vi "configRead.vi"(10 "Self":T1={"refDes"="ERR000", "IP"="localhost", "DI"=0, "DO"=0, "AI"=0, "AO"=0, "Description"="ERR", "TC"=0, "channelDefinitions"=[]}, 11 "configPath":path=path "C:/Users/miles/OneDrive - Embry-Riddle Aeronautical University/Admin/Facilities/TC3/TC3 DAC/Code/Sandbox/Node based/controlNode/Configuration/nodeConfig_0.xlsx") -> (2 "Self":T1={"refDes"="ERR000", "IP"="localhost", "DI"=0, "DO"=0, "AI"=0, "AO"=0, "Description"="ERR", "TC"=0, "channelDefinitions"=[]}, 3 "Cancel/Err":bool)   [LabVIEW 2024]
uses:
  controls/self.ctl
  controls/channelDefinition.ctl
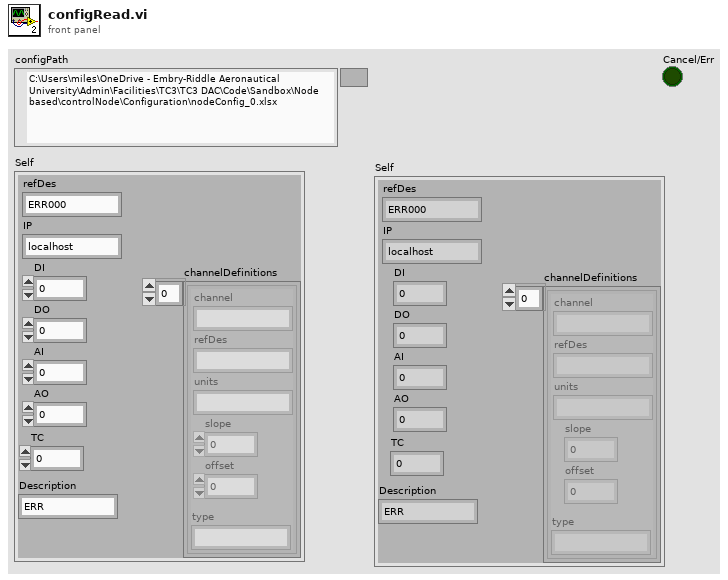
[diagram p1: front panel]
types:
  T1 = typedef "self.ctl" = cluster{"refDes":string, "IP":string, "DI":i32, "DO":i32, "AI":i32, "AO":i32, "Description":string, "TC":i32, "channelDefinitions":T2[]}
  T2 = typedef "channelDefinition.ctl" = cluster{"channel":string, "refDes":string, "units":string, "slope":dbl, "offset":dbl, "type":string}
  T3 = cluster{"[0]":string, "[1]":string, "[2]":string, "[3]":string, "[4]":string, "[5]":string, "[6]":string, "[7]":string, "[8]":string}
  T4 = cluster{"[0]":i32, "[1]":i32, "[2]":i32, "[3]":i32, "[4]":i32, "[5]":i32, "[6]":i32, "[7]":i32, "[8]":i32}
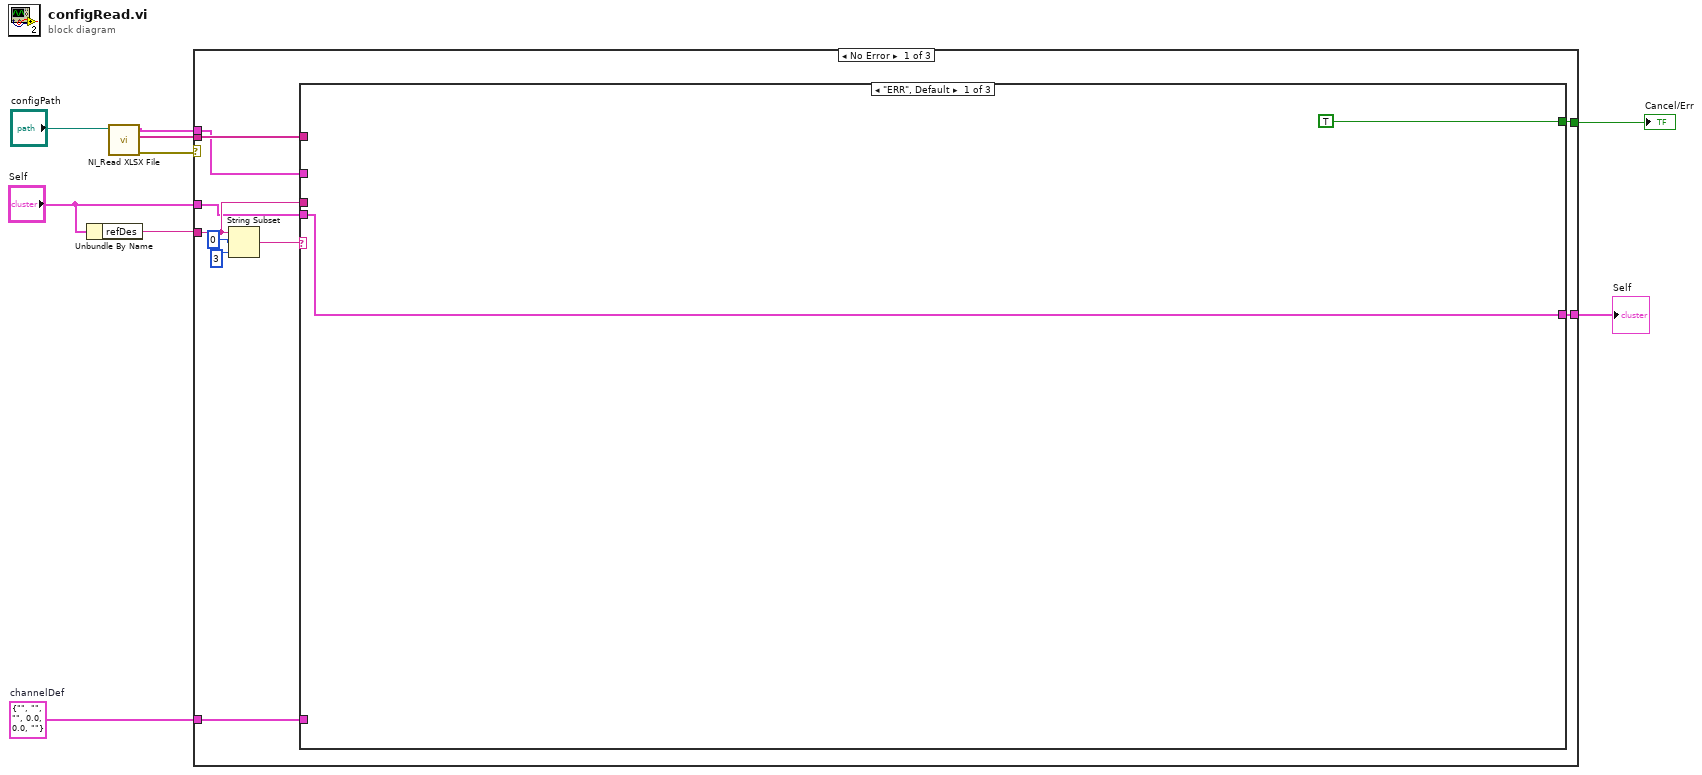
[diagram p0: block diagram]
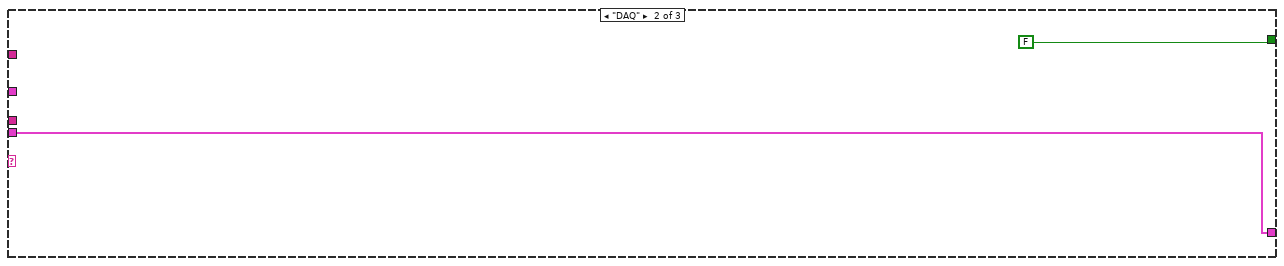
[diagram p2: hidden frame]
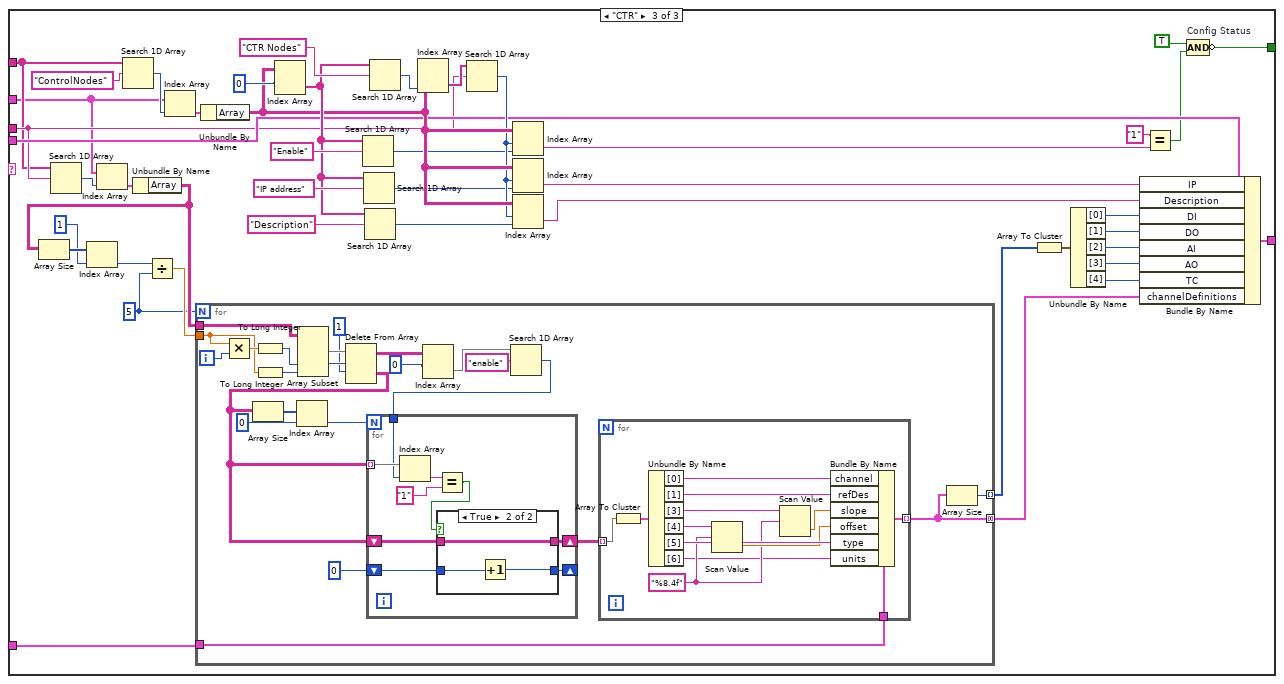
[diagram p3: hidden frame]
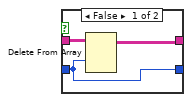
[diagram p4: hidden frame]
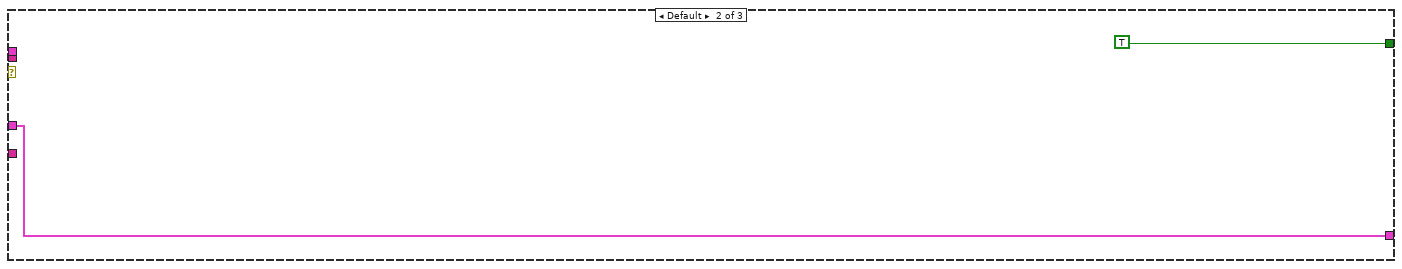
[diagram p5: hidden frame]
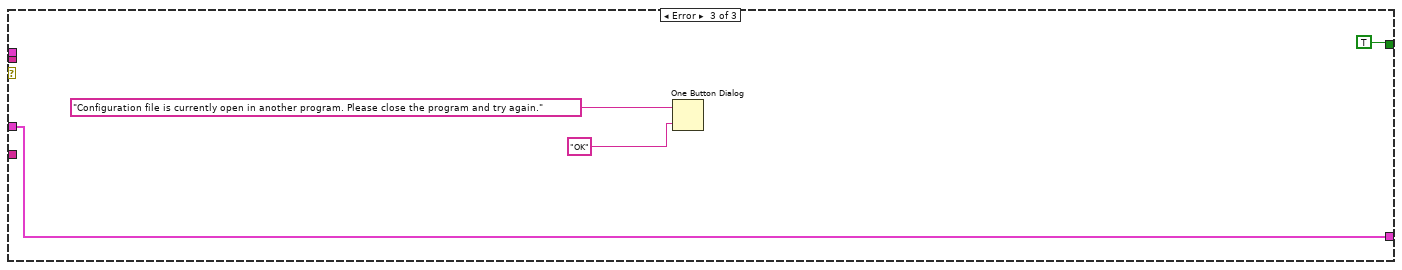
[diagram p6: hidden frame]
diagram:
  w1 = T2 {"channel"="", "refDes"="", "units"="", "slope"=0.0, "offset"=0.0, "type"=""}  # channelDef
  n1 = Unbundle By Name("Self") -> ("refDes"=w4:string)
  n2 = call "NI_Read XLSX File.vi"("XLSX File"="configPath") -> ("error out"=w8:errorcluster, "Sheet Names"=w7:string[], "Sheet Data"=w6:cluster{"Array":string[][]}[])  [unwired: 8 in]
  n3 = case shown="No Error" w8 {
    tunnel: [w13 TRUE TRUE] -> w9
    tunnel: w7 -> [w16 _ _]
    tunnel: w6 -> [w15 _ _]
    tunnel: w4 -> [w14 _ _]
    tunnel: "Self" -> [w12 w119 w123]
    tunnel: [w11 w119 w123] -> w2
    tunnel: w1 -> [w10 _ _]
    frame No Error {
      n4 = String Subset(string=w14, offset (0)=0, length (rest)=3 ("length (rest)")) -> (substring=w17:string)
      n5 = case shown="\"ERR\", Default" w17 {
        tunnel: w16 -> [_ _ w40]
        tunnel: w15 -> [_ _ w39]
        tunnel: w14 -> [_ _ w41]
        tunnel: [TRUE FALSE w60] -> w13
        tunnel: w12 -> [w20 w22 w50]
        tunnel: [w20 w22 w47] -> w11
        tunnel: w10 -> [_ _ w33]
        frame "ERR", Default {
        }
        frame "DAQ" {
        }
        frame "CTR" {
          w34 = 5 ("y")
          n6 = Search 1D Array(1D array=w40, element=w41) -> (index of element=w43:i32)  [unwired: 1 in]
          n7 = Index Array(array=w39, index=w43) -> (element=w42:cluster{"Array":string[][]})
          n8 = Search 1D Array(1D array=w40, element="ControlNodes") -> (index of element=w67:i32)  [unwired: 1 in]
          n9 = Unbundle By Name(w42) -> ("Array"=w38:string[][])
          n10 = Array Size(array=w38) -> (size(s)=w37:i32[])
          n11 = Index Array(array=w37, index=1) -> (element=w24:i32)
          n12 = Divide(x=w24, y=w34) -> (x/y=w35:dbl)
          n13 = Index Array(array=w39, index=w67) -> (element=w66:cluster{"Array":string[][]})
          n14 = for {
            N: w34 -> [_]
            tunnel: w38 -> [w90]
            tunnel: w35 -> [w88]
            tunnel: w33 -> [w78]
            tunnel: [w77] -> w25 mode=concatenating
            tunnel: [w76] -> w32 mode=indexing
            i -> [w75]
            n15 = Multiply(x=w88, y=w75) -> (x*y=w89:dbl)
            n16 = To Long Integer(number=w89) -> (32bit integer=w87:i32)
            n17 = To Long Integer(number=w88) -> (32bit integer=w85:i32)
            n18 = Array Subset(array=w90, index (col)=w87, length (col)=w85) -> (w86:string[][])  [unwired: 2 in]
            n19 = Delete From Array(array=w86, length=w85, index (row)=1) -> (deleted portion=w80:string[][], array with subset deleted=w71:string[][])  [unwired: 1 in]
            n20 = Array Size(array=w80) -> (size(s)=w84:i32[])
            n21 = Index Array(array=w84, index=0) -> (element=w82:i32)
            n22 = Index Array(array=w71, index (row)=0) -> (element=w73:string[])  [unwired: 1 in]
            n23 = Search 1D Array(1D array=w73, element="enable") -> (index of element=w70:i32)  [unwired: 1 in]
            n24 = for {
              N: w82 -> [_]
              tunnel: w80 -> [w110] mode=indexing
              shift-right: [w107] -> w79
              shift-left: w80 -> [w109]
              tunnel: w70 -> [w106]
              shift-right: [w104] -> _
              shift-left: 0 -> [w105]
              n25 = Index Array(array=w110, index=w106) -> (element=w112:string)
              n26 = Equal?(x=w112, y="1") -> (x = y?=w108:bool)
              n27 = case shown="True" w108 {
                tunnel: w109 -> [w115 w118]
                tunnel: [w114 w118] -> w107
                tunnel: w105 -> [w113 w117]
                tunnel: [w113 w116] -> w104
                frame False {
                  n28 = Delete From Array(array=w115, index (row)=w113) -> (array with subset deleted=w114:string[][])  [unwired: 2 in, 1 out]
                }
                frame True {
                  n29 = Increment(x=w117) -> (x+1=w116:i32)
                }
              }
            }
            n30 = for {
              tunnel: w79 -> [w94] mode=indexing
              tunnel: w78 -> [w93]
              tunnel: [w92] -> w77 mode=indexing
              w95 = "%8.4f"
              n31 = Array To Cluster(array=w94) -> (cluster=w103:T3)
              n32 = Unbundle By Name(w103) -> ("[0]"=w102:string, "[1]"=w101:string, "[3]"=w99:string, "[4]"=w97:string, "[5]"=w100:string, "[6]"=w91:string)
              n33 = Scan Value(string=w97, format string=w95) -> (value=w96:dbl)  [unwired: 1 in, 1 out]
              n34 = Scan Value(string=w99, format string=w95) -> (value=w98:dbl)  [unwired: 1 in, 1 out]
              n35 = Bundle By Name(cluster=w93, "channel"=w102, "refDes"=w101, "slope"=w98, "offset"=w96, "type"=w100, "units"=w91) -> (w92:T2)
            }
            n36 = Array Size(array=w77) -> (size(s)=w76:i32)
          }
          n37 = Unbundle By Name(w66) -> ("Array"=w55:string[][])
          n38 = Index Array(array=w55, index (row)=0) -> (element=w56:string[])  [unwired: 1 in]
          n39 = Search 1D Array(1D array=w56, element="Enable") -> (index of element=w53:i32)  [unwired: 1 in]
          n40 = Search 1D Array(1D array=w56, element="IP address") -> (index of element=w52:i32)  [unwired: 1 in]
          n41 = Search 1D Array(1D array=w56, element="Description") -> (index of element=w51:i32)  [unwired: 1 in]
          n42 = Search 1D Array(1D array=w56, element="CTR Nodes") -> (index of element=w63:i32)  [unwired: 1 in]
          n43 = Index Array(array=w55, index (col)=w63) -> (element=w62:string[])  [unwired: 1 in]
          n44 = Search 1D Array(1D array=w62, element=w41) -> (index of element=w54:i32)  [unwired: 1 in]
          n45 = Index Array(array=w55, index (row)=w54, index (col)=w53) -> (element=w45:string)
          n46 = Index Array(array=w55, index (row)=w54, index (col)=w52) -> (element=w49:string)
          n47 = Index Array(array=w55, index (row)=w54, index (col)=w51) -> (element=w48:string)
          n48 = Array To Cluster(array=w32) -> (cluster=w31:T4)
          n49 = Unbundle By Name(w31) -> ("[0]"=w30:i32, "[1]"=w29:i32, "[2]"=w28:i32, "[3]"=w27:i32, "[4]"=w26:i32)
          n50 = Bundle By Name(cluster=w50, "IP"=w49, "Description"=w48, "DI"=w30, "DO"=w29, "AI"=w28, "AO"=w27, "TC"=w26, "channelDefinitions"=w25) -> (w47:T1)
          n51 = Equal?(x="1", y=w45) -> (x = y?=w44:bool)
          n52 = Compound Arithmetic op=AND "Config Status"(TRUE, w44) -> (invert w60:bool)
        }
      }
    }
    frame Default {
    }
    frame Error {
      n53 = One Button Dialog(message="Configuration file is currently open in another program. Please close the program and try again.", button name ("OK")="OK") -> ()  [unwired: 1 out]
    }
  }
  "Cancel/Err" <- w9
  "Self" <- w2
